vi "Prog5.vi"() -> ()   [LabVIEW 2021]
panel:
  out "unsigned byte array 3":u8[](array[numeric])
  out "unsigned byte array 7":u8[](array[numeric])
  out "unsigned byte array 6":u8[](array[numeric])
  out "unsigned byte array 5":u8[](array[numeric])
  out "unsigned byte array 4":u8[](array[numeric])
  out "unsigned byte array 2":u8[](array[numeric])
  out "unsigned byte array":u8[](array[numeric])
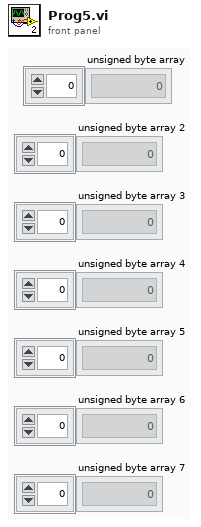
[diagram p1: front panel]
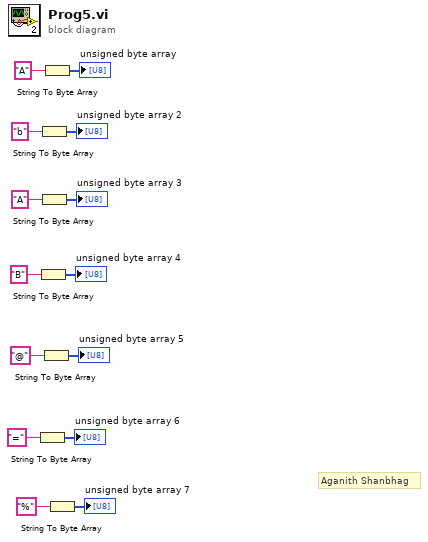
[diagram p0: block diagram]
diagram:
  # "Aganith Shanbhag"
  n1 = String To Byte Array(string="=") -> (unsigned byte array=→"unsigned byte array 6":u8[])
  n2 = String To Byte Array(string="B") -> (unsigned byte array=→"unsigned byte array 4":u8[])
  n3 = String To Byte Array(string="b") -> (unsigned byte array=→"unsigned byte array 2":u8[])
  n4 = String To Byte Array(string="A") -> (unsigned byte array=→"unsigned byte array 3":u8[])
  n5 = String To Byte Array(string="@") -> (unsigned byte array=→"unsigned byte array 5":u8[])
  n6 = String To Byte Array(string="A") -> (unsigned byte array=→"unsigned byte array":u8[])
  n7 = String To Byte Array(string="%") -> (unsigned byte array=→"unsigned byte array 7":u8[])
